vi "Do.vi"(8 "error in (no error)":errorcluster, 10 "Actor in":refnum<class "Actor.lvclass">, 11 "UnregisterAppenderMsg":refnum<class "UnregisterAppenderMsg.lvclass">) -> (0 "error out":errorcluster, 2 "Actor out":refnum<class "Actor.lvclass">)   [LabVIEW 2026, in "Lumberjack.lvlib" / "UnregisterAppenderMsg.lvclass"]
doc: "<p>(<strong>Filename</strong>: <span class=\"dnl\">Actor Framework.lvlib:Message.lvclass:Do.vi</span>)</p>\n<p>Defines what a message does when it is received by an actor. Generally, a message instructs an actor to invoke one of its methods. By default, this method does nothing. A child class must override it to define behavior.</p>"
uses:
  UnregisterAppenderMsg.lvclass
  <vilib>/ActorFramework/Actor/Actor.lvclass
  LogManager/LogManager.lvclass/LogManager.lvclass
  UnregisterAppenderMsg.lvclass/UnregisterAppenderMsg.ctl
  <vilib>/ActorFramework/Message Enqueuer/Message Enqueuer.lvclass/Message Enqueuer.ctl
  <vilib>/ActorFramework/Message Enqueuer/Enqueue.vi
  <vilib>/ActorFramework/Stop Msg/Stop Msg.lvclass
  <vilib>/ActorFramework/Message Priority Queue/Priority Enqueue.vi
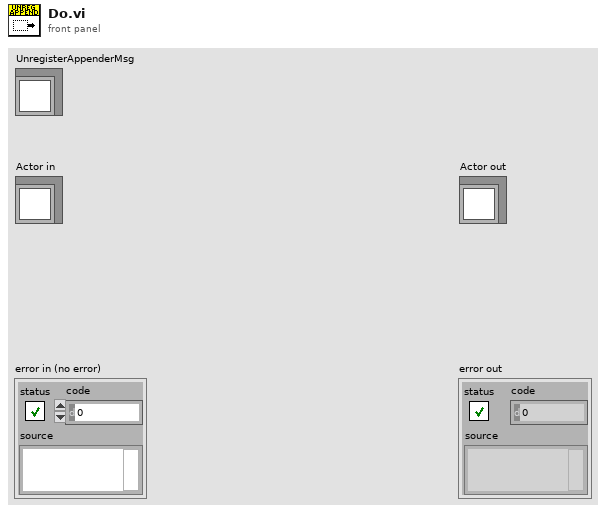
[diagram p1: front panel]
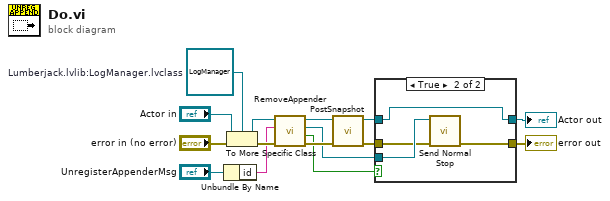
[diagram p0: block diagram]
diagram:
  w10 = refnum<class "LogManager.lvclass"> refnum  # Lumberjack.lvlib:LogManager.lvclass
  n1 = Unbundle By Name("UnregisterAppenderMsg") -> ("id"=w8:string)
  n2 = To More Specific Class(target class=w10, reference="Actor in", error in="error in (no error)") -> (specific class reference=w7:refnum<class "LogManager.lvclass">, error out=w9:errorcluster)
  n3 = call "RemoveAppender.vi"("error in (no error)"=w9, "id"=w8, "LogManager in"=w7) -> ("error out"=w14:errorcluster, "found"=w5:bool, "removedEnqueuer"=w6:refnum<class "Message Enqueuer.lvclass">, "LogManager out"=w15:refnum<class "LogManager.lvclass">)  [unwired: 5 in]
  n4 = call "PostSnapshot.vi"("error in (no error)"=w14, "LogManager in"=w15) -> ("error out"=w4:errorcluster, "LogManager out"=w3:refnum<class "LogManager.lvclass">)  [unwired: 8 in]
  n5 = case shown="True" w5 {
    tunnel: w6 -> [_ w21]
    tunnel: w4 -> [w17 w20]
    tunnel: w3 -> [w16 w18]
    tunnel: [w17 w19] -> w2
    tunnel: [w16 w18] -> w1
    frame False {
    }
    frame True {
      n6 = call <vilib>:"Send Normal Stop.vi"("error in (no error)"=w20, "Message Enqueuer"=w21) -> ("error out"=w19:errorcluster)  [unwired: 9 in]
    }
  }
  "error out" <- w2
  "Actor out" <- w1
